vi "Set Tree Refnum.vi"(8 "error in (no error)":errorcluster, 10 "Tree":refnum<vi>, 11 "TREE in":refnum<class "MyTreeAPI.lvclass">) -> (0 "error out":errorcluster, 3 "TREE out":refnum<class "MyTreeAPI.lvclass">)   [LabVIEW 2015, in "MyTreeAPI.lvclass"]
uses:
  MyTreeAPI.lvclass
  MyTreeAPI.lvclass/MyTreeAPI.ctl
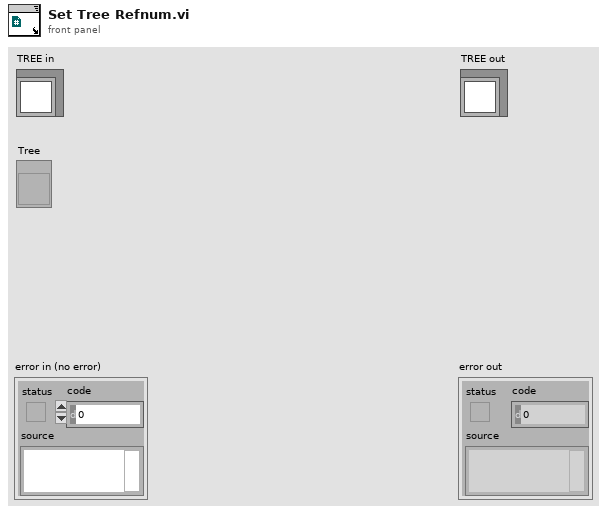
[diagram p1: front panel]
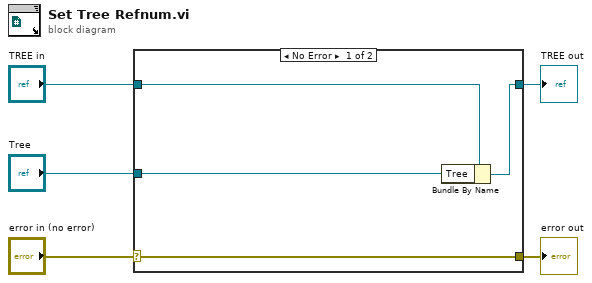
[diagram p0: block diagram]
diagram:
  n1 = case shown="No Error" "error in (no error)" {
    selector: "error in (no error)" -> [w9 w10]
    tunnel: [w9 w10] -> w4
    tunnel: [w7 w11] -> w2
    tunnel: "TREE in" -> [w8 w11]
    tunnel: "Tree" -> [w6 _]
    frame No Error {
      n2 = Bundle By Name(cluster=w8, "Tree"=w6) -> (w7:refnum<class "MyTreeAPI.lvclass">)
    }
    frame Error {
    }
  }
  "error out" <- w4
  "TREE out" <- w2
